vi "Calc - B.vi"(9 "P1":dbl, 10 "P2":dbl, 11 "Y1":dbl) -> (3 "B":dbl)   [LabVIEW 2018, in "Controller (Host).lvlib"]
uses:
  Controller (Host).lvlib
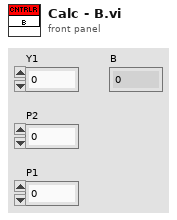
[diagram p1: front panel]
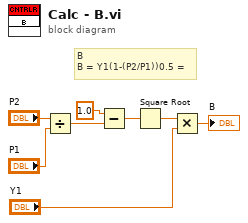
[diagram p0: block diagram]
diagram:
  # "B \nB = Y1(1-(P2/P1))0.5 ="
  n1 = Divide(x="P2", y="P1") -> (x/y=w3:dbl)
  n2 = Subtract(x=1.0, y=w3) -> (x-y=w4:dbl)
  n3 = Square Root(x=w4) -> (sqrt(x)=w1:dbl)
  n4 = Multiply(x=w1, y="Y1") -> (x*y=→"B":dbl)
